vi "HandlePauseSync.vi"(8 "error in (no error)":errorcluster, 11 "S4GUI in":refnum<class "S4GUI.lvclass">) -> (0 "error out":errorcluster, 3 "S4GUI out":refnum<class "S4GUI.lvclass">)   [LabVIEW 2018, in "S4GUI.lvclass"]
uses:
  S4GUI.lvclass
  S4GUI.lvclass/S4GUI.ctl
  Acquisition/Acquisition.lvclass
  Channel/Channel.lvclass
  StateMachine/State Machine.lvclass
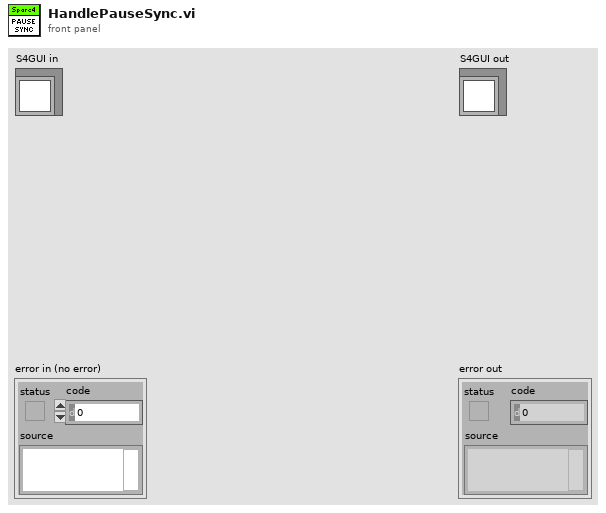
[diagram p1: front panel]
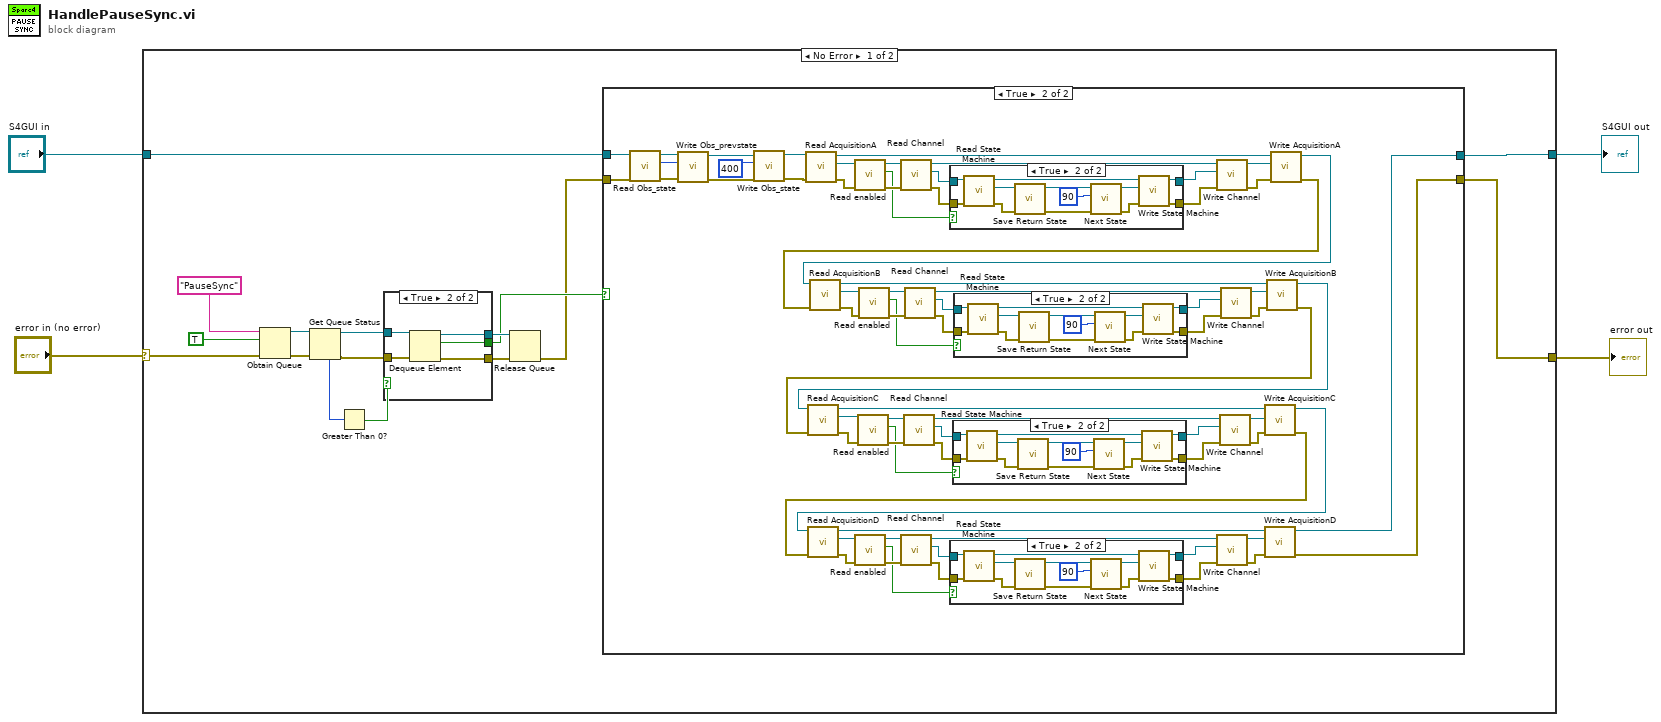
[diagram p0: block diagram]
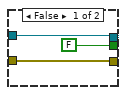
[diagram p2: hidden frame]
diagram:
  n1 = case shown="No Error" "error in (no error)" {
    selector: "error in (no error)" -> [w7 w158]
    tunnel: [w5 w158] -> w3
    tunnel: [w6 w157] -> w1
    tunnel: "S4GUI in" -> [w8 w157]
    frame No Error {
      n2 = Obtain Queue(name (unnamed)="PauseSync", element data type=TRUE, error in (no error)=w7) -> (queue out=w17:refnum<queue>, error out=w18:errorcluster)  [unwired: 2 in, 1 out]
      n3 = Get Queue Status(queue=w17, error in (no error)=w18) -> (queue out=w14:refnum<queue>, error out=w13:errorcluster, # elements in queue=w16:i32)  [unwired: 1 in, 5 out]
      n4 = Greater Than 0?(x=w16) -> (x > 0?=w15:bool)
      n5 = case shown="True" w15 {
        tunnel: w14 -> [w22 w27]
        tunnel: w13 -> [w21 w28]
        tunnel: [FALSE w26] -> w10
        tunnel: [w22 w25] -> w12
        tunnel: [w21 w24] -> w11
        frame False {
        }
        frame True {
          n6 = Dequeue Element(queue=w27, error in (no error)=w28) -> (queue out=w25:refnum<queue>, element=w26:bool, error out=w24:errorcluster)  [unwired: 1 in, 1 out]
        }
      }
      n7 = Release Queue(queue=w12, error in (no error)=w11) -> (error out=w9:errorcluster)  [unwired: 1 in, 2 out]
      n8 = case shown="True" w10 {
        tunnel: w9 -> [w29 w93]
        tunnel: w8 -> [w30 w94]
        tunnel: [w30 w74] -> w6
        tunnel: [w29 w78] -> w5
        frame False {
        }
        frame True {
          n9 = call-dynamic "Read Obs_state.vi"("error in (no error)"=w93, "S4ACS_GUI in"=w94) -> ("error out"=w98:errorcluster, "Obs_state"=w100:u32, "S4ACS_GUI out"=w99:refnum<class "S4GUI.lvclass">)  [unwired: 7 in]
          n10 = call-dynamic "Write Obs_prevstate.vi"("error in (no error)"=w98, "Obs_prevstate"=w100, "S4ACS_GUI in"=w99) -> ("error out"=w96:errorcluster, "S4ACS_GUI out"=w97:refnum<class "S4GUI.lvclass">)  [unwired: 7 in]
          n11 = call-dynamic "Write Obs_state.vi"("error in (no error)"=w96, "Obs_state"=u32 400, "S4ACS_GUI in"=w97) -> ("error out"=w91:errorcluster, "S4ACS_GUI out"=w92:refnum<class "S4GUI.lvclass">)  [unwired: 7 in]
          n12 = call-dynamic "Read AcquisitionA.vi"("error in (no error)"=w91, "S4ACS_GUI in"=w92) -> ("error out"=w72:errorcluster, "Acquisition.lvclass"=w73:refnum<class "Acquisition.lvclass">, "S4ACS_GUI out"=w90:refnum<class "S4GUI.lvclass">)  [unwired: 7 in]
          n13 = call-dynamic "Read enabled.vi"("error in (no error)"=w72, "Server in"=w73) -> ("error out"=w70:errorcluster, "enabled"=w67:bool, "Server out"=w71:refnum<class "Acquisition.lvclass">)  [unwired: 7 in]
          n14 = call-dynamic "Read Channel.vi"("error in (no error)"=w70, "Acquisition in"=w71) -> ("error out"=w68:errorcluster, "Channel.lvclass"=w69:refnum<class "Channel.lvclass">, "Acquisition out"=w89:refnum<class "Acquisition.lvclass">)  [unwired: 7 in]
          n15 = case shown="True" w67 {
            tunnel: w69 -> [w144 w156]
            tunnel: [w144 w154] -> w87
            tunnel: w68 -> [w143 w149]
            tunnel: [w143 w145] -> w86
            frame False {
            }
            frame True {
              n16 = call-dynamic "Read State Machine.vi"("error in (no error)"=w149, "Device in"=w156) -> ("error out"=w148:errorcluster, "State Machine.lvclass"=w153:refnum<class "State Machine.lvclass">, "Device out"=w155:refnum<class "Channel.lvclass">)  [unwired: 7 in]
              n17 = call-dynamic "Save Return State.vi"("error in (no error)"=w148, "State Machine in"=w153) -> ("error out"=w147:errorcluster, "State Machine out"=w152:refnum<class "State Machine.lvclass">)  [unwired: 8 in]
              n18 = call "Next State.vi"("error in (no error)"=w147, "New_State"=90, "State Machine in"=w152) -> ("error out"=w146:errorcluster, "State Machine out"=w151:refnum<class "State Machine.lvclass">)  [unwired: 7 in]
              n19 = call-dynamic "Write State Machine.vi"("error in (no error)"=w146, "State Machine.lvclass"=w151, "Device in"=w155) -> ("error out"=w145:errorcluster, "Device out"=w154:refnum<class "Channel.lvclass">)  [unwired: 7 in]
            }
          }
          n20 = call-dynamic "Write Channel.vi"("error in (no error)"=w86, "Channel.lvclass"=w87, "Acquisition in"=w89) -> ("error out"=w85:errorcluster, "Acquisition out"=w88:refnum<class "Acquisition.lvclass">)  [unwired: 7 in]
          n21 = call-dynamic "Write AcquisitionA.vi"("error in (no error)"=w85, "Acquisition.lvclass"=w88, "S4ACS_GUI in"=w90) -> ("error out"=w81:errorcluster, "S4ACS_GUI out"=w77:refnum<class "S4GUI.lvclass">)  [unwired: 7 in]
          n22 = call "Read AcquisitionB.vi"("error in (no error)"=w81, "S4ACS_GUI in"=w77) -> ("error out"=w57:errorcluster, "Acquisition.lvclass"=w58:refnum<class "Acquisition.lvclass">, "S4ACS_GUI out"=w84:refnum<class "S4GUI.lvclass">)  [unwired: 7 in]
          n23 = call-dynamic "Read enabled.vi"("error in (no error)"=w57, "Server in"=w58) -> ("error out"=w62:errorcluster, "enabled"=w59:bool, "Server out"=w63:refnum<class "Acquisition.lvclass">)  [unwired: 7 in]
          n24 = call-dynamic "Read Channel.vi"("error in (no error)"=w62, "Acquisition in"=w63) -> ("error out"=w60:errorcluster, "Channel.lvclass"=w61:refnum<class "Channel.lvclass">, "Acquisition out"=w66:refnum<class "Acquisition.lvclass">)  [unwired: 7 in]
          n25 = case shown="True" w59 {
            tunnel: w61 -> [w130 w142]
            tunnel: [w130 w140] -> w65
            tunnel: w60 -> [w129 w135]
            tunnel: [w129 w131] -> w64
            frame False {
            }
            frame True {
              n26 = call-dynamic "Read State Machine.vi"("error in (no error)"=w135, "Device in"=w142) -> ("error out"=w134:errorcluster, "State Machine.lvclass"=w139:refnum<class "State Machine.lvclass">, "Device out"=w141:refnum<class "Channel.lvclass">)  [unwired: 7 in]
              n27 = call-dynamic "Save Return State.vi"("error in (no error)"=w134, "State Machine in"=w139) -> ("error out"=w133:errorcluster, "State Machine out"=w138:refnum<class "State Machine.lvclass">)  [unwired: 8 in]
              n28 = call "Next State.vi"("error in (no error)"=w133, "New_State"=90, "State Machine in"=w138) -> ("error out"=w132:errorcluster, "State Machine out"=w137:refnum<class "State Machine.lvclass">)  [unwired: 7 in]
              n29 = call-dynamic "Write State Machine.vi"("error in (no error)"=w132, "State Machine.lvclass"=w137, "Device in"=w141) -> ("error out"=w131:errorcluster, "Device out"=w140:refnum<class "Channel.lvclass">)  [unwired: 7 in]
            }
          }
          n30 = call-dynamic "Write Channel.vi"("error in (no error)"=w64, "Channel.lvclass"=w65, "Acquisition in"=w66) -> ("error out"=w55:errorcluster, "Acquisition out"=w56:refnum<class "Acquisition.lvclass">)  [unwired: 7 in]
          n31 = call "Write AcquisitionB.vi"("error in (no error)"=w55, "Acquisition.lvclass"=w56, "S4ACS_GUI in"=w84) -> ("error out"=w80:errorcluster, "S4ACS_GUI out"=w76:refnum<class "S4GUI.lvclass">)  [unwired: 7 in]
          n32 = call-dynamic "Read AcquisitionC.vi"("error in (no error)"=w80, "S4ACS_GUI in"=w76) -> ("error out"=w44:errorcluster, "Acquisition.lvclass"=w46:refnum<class "Acquisition.lvclass">, "S4ACS_GUI out"=w83:refnum<class "S4GUI.lvclass">)  [unwired: 7 in]
          n33 = call-dynamic "Read enabled.vi"("error in (no error)"=w44, "Server in"=w46) -> ("error out"=w50:errorcluster, "enabled"=w47:bool, "Server out"=w51:refnum<class "Acquisition.lvclass">)  [unwired: 7 in]
          n34 = call-dynamic "Read Channel.vi"("error in (no error)"=w50, "Acquisition in"=w51) -> ("error out"=w48:errorcluster, "Channel.lvclass"=w49:refnum<class "Channel.lvclass">, "Acquisition out"=w54:refnum<class "Acquisition.lvclass">)  [unwired: 7 in]
          n35 = case shown="True" w47 {
            tunnel: w49 -> [w116 w128]
            tunnel: [w116 w126] -> w53
            tunnel: w48 -> [w115 w121]
            tunnel: [w115 w117] -> w52
            frame False {
            }
            frame True {
              n36 = call-dynamic "Read State Machine.vi"("error in (no error)"=w121, "Device in"=w128) -> ("error out"=w120:errorcluster, "State Machine.lvclass"=w125:refnum<class "State Machine.lvclass">, "Device out"=w127:refnum<class "Channel.lvclass">)  [unwired: 7 in]
              n37 = call-dynamic "Save Return State.vi"("error in (no error)"=w120, "State Machine in"=w125) -> ("error out"=w119:errorcluster, "State Machine out"=w124:refnum<class "State Machine.lvclass">)  [unwired: 8 in]
              n38 = call "Next State.vi"("error in (no error)"=w119, "New_State"=90, "State Machine in"=w124) -> ("error out"=w118:errorcluster, "State Machine out"=w123:refnum<class "State Machine.lvclass">)  [unwired: 7 in]
              n39 = call-dynamic "Write State Machine.vi"("error in (no error)"=w118, "State Machine.lvclass"=w123, "Device in"=w127) -> ("error out"=w117:errorcluster, "Device out"=w126:refnum<class "Channel.lvclass">)  [unwired: 7 in]
            }
          }
          n40 = call-dynamic "Write Channel.vi"("error in (no error)"=w52, "Channel.lvclass"=w53, "Acquisition in"=w54) -> ("error out"=w43:errorcluster, "Acquisition out"=w45:refnum<class "Acquisition.lvclass">)  [unwired: 7 in]
          n41 = call-dynamic "Write AcquisitionC.vi"("error in (no error)"=w43, "Acquisition.lvclass"=w45, "S4ACS_GUI in"=w83) -> ("error out"=w79:errorcluster, "S4ACS_GUI out"=w75:refnum<class "S4GUI.lvclass">)  [unwired: 7 in]
          n42 = call-dynamic "Read AcquisitionD.vi"("error in (no error)"=w79, "S4ACS_GUI in"=w75) -> ("error out"=w33:errorcluster, "Acquisition.lvclass"=w34:refnum<class "Acquisition.lvclass">, "S4ACS_GUI out"=w82:refnum<class "S4GUI.lvclass">)  [unwired: 7 in]
          n43 = call-dynamic "Read enabled.vi"("error in (no error)"=w33, "Server in"=w34) -> ("error out"=w38:errorcluster, "enabled"=w35:bool, "Server out"=w39:refnum<class "Acquisition.lvclass">)  [unwired: 7 in]
          n44 = call-dynamic "Read Channel.vi"("error in (no error)"=w38, "Acquisition in"=w39) -> ("error out"=w36:errorcluster, "Channel.lvclass"=w37:refnum<class "Channel.lvclass">, "Acquisition out"=w42:refnum<class "Acquisition.lvclass">)  [unwired: 7 in]
          n45 = case shown="True" w35 {
            tunnel: w37 -> [w102 w114]
            tunnel: [w102 w112] -> w41
            tunnel: w36 -> [w101 w107]
            tunnel: [w101 w103] -> w40
            frame False {
            }
            frame True {
              n46 = call-dynamic "Read State Machine.vi"("error in (no error)"=w107, "Device in"=w114) -> ("error out"=w106:errorcluster, "State Machine.lvclass"=w111:refnum<class "State Machine.lvclass">, "Device out"=w113:refnum<class "Channel.lvclass">)  [unwired: 7 in]
              n47 = call-dynamic "Save Return State.vi"("error in (no error)"=w106, "State Machine in"=w111) -> ("error out"=w105:errorcluster, "State Machine out"=w110:refnum<class "State Machine.lvclass">)  [unwired: 8 in]
              n48 = call "Next State.vi"("error in (no error)"=w105, "New_State"=90, "State Machine in"=w110) -> ("error out"=w104:errorcluster, "State Machine out"=w109:refnum<class "State Machine.lvclass">)  [unwired: 7 in]
              n49 = call-dynamic "Write State Machine.vi"("error in (no error)"=w104, "State Machine.lvclass"=w109, "Device in"=w113) -> ("error out"=w103:errorcluster, "Device out"=w112:refnum<class "Channel.lvclass">)  [unwired: 7 in]
            }
          }
          n50 = call-dynamic "Write Channel.vi"("error in (no error)"=w40, "Channel.lvclass"=w41, "Acquisition in"=w42) -> ("error out"=w32:errorcluster, "Acquisition out"=w31:refnum<class "Acquisition.lvclass">)  [unwired: 7 in]
          n51 = call-dynamic "Write AcquisitionD.vi"("error in (no error)"=w32, "Acquisition.lvclass"=w31, "S4ACS_GUI in"=w82) -> ("error out"=w78:errorcluster, "S4ACS_GUI out"=w74:refnum<class "S4GUI.lvclass">)  [unwired: 7 in]
        }
      }
    }
    frame Error {
    }
  }
  "error out" <- w3
  "S4GUI out" <- w1
